vi "Lab Panel V5.0.vi"() -> ()   [LabVIEW 2013] (continued)
                        w1540 = "\\"
                        n878 = local read "SET LAB05-1"() -> (w1548:T5)
                        n879 = case shown="\"CYCLE TEST\"" w1553 {
                          tunnel: ["L05-1-CHART TEST-" "L05-1-CYCLE TEST-" "L05-1-T-RISE TEST-"] -> w1549
                          frame "CHART TEST", Default {
                          }
                          frame "CYCLE TEST" {
                          }
                          frame "T-RISE TEST" {
                          }
                        }
                        n880 = Unbundle(w1548) -> ("DESCRIPTION"=w1547:string)  [unwired: 4 out]
                        n881 = Concatenate Strings(w1543, "\\", w1541, w1540, w1539, w1540) -> (w1550:string)
                        n882 = String To Path(string=w1550) -> (path=w1552:path)
                        n883 = Concatenate Strings(w1550, w1549, w1547, "-", w1546, ".tdms") -> (w1538:string)
                        n884 = Create Folder(path (use dialog)=w1552) -> (error out=w1551:errorcluster)  [unwired: 2 in, 2 out]
                        n885 = global write "Global 1.vi" "LAB05-1 FILE"(w1538) -> ()
                        n886 = call <vilib>:"Clear Errors.vi"("error in (no error)"=w1551) -> ()  [unwired: 6 in, 1 out]
                      }
                      frame #1 {
                        (unwired) FALSE
                        n887 = String To Path(string=w1562) -> (path=w1558:path)
                        n888 = TDMS Open(6:FALSE, 10:T18."create or replace" ("operation (0:open)"), 11:w1558) -> (0:w1557:errorcluster, 3:→"TDMS LAB05-1":refnum<k34>)  [unwired: 4 in]
                      }
                      frame #2 {
                        n889 = local read "SET LAB05-1"() -> (w1568:T5)
                        n890 = local read "TDMS LAB05-1"() -> (w1579:refnum<k34>)
                        n891 = Build Array("Testers Name", "Description", "Set Test Cycles", "T-Rise minutes", "T-Rise Deg C") -> (w1569:string[])
                        n892 = Unbundle(w1568) -> ("NAME"=w1567:string, "DESCRIPTION"=w1566:string, "CYCLES"=w1565:dbl, "T-RISE mins"=w1564:dbl, "T-RISE deg C"=w1563:dbl)
                        n893 = Number To Decimal String(number=w1565) -> (decimal integer string=w1578:string)  [unwired: 1 in]
                        n894 = Number To Decimal String(number=w1564) -> (decimal integer string=w1577:string)  [unwired: 1 in]
                        n895 = Number To Decimal String(number=w1563) -> (decimal integer string=w1576:string)  [unwired: 1 in]
                        n896 = Build Array(w1567, w1566, w1578, w1577, w1576) -> (w1575:string[])
                        n897 = TDMS Set Properties(5:w1575, 7:w1569, 11:w1579) -> ()  [unwired: 3 in, 4 out]
                      }
                      frame #3 {
                        n898 = local read "DISP LAB05-1"() -> (w1584:T4)
                        n899 = Concatenate Strings("LAB05-1  ", w1582) -> (w1585:string)
                        n900 = Two Button Dialog(message=w1585, 1:w1580, 2:w1581) -> (T button?=w1587:bool)
                        n901 = case shown="True" w1587 {
                          tunnel: w1584 -> [w1594 w1595]
                          tunnel: [w1594 w1595] -> w1591
                          tunnel: [w1593 w1596] -> w1590
                          tunnel: [w1592 w1596] -> w1589
                          frame False {
                            n902 = Unbundle(w1594) -> ("CYCLE"=w1593:dbl, "MINS"=w1592:dbl)  [unwired: 1 out]
                          }
                          frame True {
                            w1596 = 0.0
                          }
                        }
                        n903 = Bundle(cluster=w1591, "CYCLE"=w1590, "MINS"=w1589, "STATUS"="RUN") -> (w1583:T4)
                        n904 = local write "DISP LAB05-1"(w1583) -> ()
                      }
                      frame #4 {
                        n905 = local read "SIG LAB05-1"() -> (w1599:T2)
                        n906 = local read "TEMP START LAB05-1"() -> (w1601:cluster{"TL":dbl, "TN":dbl})
                        n907 = Unbundle(w1599) -> ("Tmp Live"=w1598:dbl, "Tmp Neut"=w1597:dbl)  [unwired: 3 out]
                        n908 = Bundle(cluster=w1601, "TL"=w1598, "TN"=w1597) -> (w1600:cluster{"TL":dbl, "TN":dbl})
                        n909 = local write "TEMP START LAB05-1"(w1600) -> ()
                      }
                    }
                  }
                }
              }
              event "RUN LAB05-2": Value Change {
                n910 = event-data() -> ("NewVal"=w1605:bool)  [unwired: 1 in, 5 out]
                n911 = local write "run lab05-2"(w1605) -> ()
                n912 = case shown="True" w1605 {
                  tunnel: w1611 -> [_ w1647]
                  tunnel: w1610 -> [_ w1646]
                  tunnel: w1608 -> [w1613 w1645]
                  tunnel: w1609 -> [_ w1644]
                  tunnel: w1607 -> [_ w1643]
                  tunnel: [w1612 w1642] -> w1606
                  tunnel: w1604 -> [_ w1641]
                  tunnel: w1603 -> [_ w1640]
                  tunnel: w1602 -> [_ w1639]
                  frame False {
                    # "stop test"
                    n913 = stacked-sequence {
                      tunnel: w1613 -> [w1622 _]
                      tunnel: [w1614 _] -> w1612
                      frame #0 {
                        n914 = local read "DISP LAB05-2"() -> (w1621:T4)
                        n915 = Unbundle(w1621) -> ("CYCLE"=w1619:dbl, "MINS"=w1620:dbl)  [unwired: 1 out]
                        n916 = case shown="\"CYCLE TEST\"" w1622 {
                          tunnel: w1620 -> [_ _ w1629]
                          tunnel: w1619 -> [w1627 w1628 _]
                          tunnel: [w1627 w1628 w1629] -> w1618
                          frame "CHART TEST", Default {
                          }
                          frame "CYCLE TEST" {
                          }
                          frame "T-RISE TEST" {
                          }
                        }
                        n917 = local read "TDMS LAB05-2"() -> (w1626:refnum<k34>)
                        n918 = Build Array("STOPPED") -> (w1623:string[])
                        n919 = Build Array(w1618) -> (w1617:dbl[])
                        n920 = TDMS Write(0:w1626, 5:"TEST RESULT", 7:w1623, 9:w1617) -> (4:w1615:refnum<k34>, 15:w1616:errorcluster)  [unwired: 2 in, 2 out]
                        n921 = TDMS Close(8:w1616, 11:w1615) -> (0:w1614:errorcluster)  [unwired: 1 out]
                      }
                      frame #1 {
                        n922 = local read "DISP LAB05-2"() -> (w1633:T4)
                        n923 = stacked-sequence {
                          tunnel: "LAB05-2" -> [w1635 w1637]
                          frame #0 {
                            n924 = call "sub vi - defrag tdms v1.vi"("panel id"=w1635) -> ("error out"=w1634:errorcluster)  [unwired: 10 in]
                            n925 = local write "data file error"(w1634) -> ()
                          }
                          frame #1 {
                            n926 = local write "RESULT LAB05-2"(FALSE) -> ()
                            n927 = call "Save data file to network drive v2.vi"("panel id"=w1637) -> ("network file save error"=w1636:errorcluster)  [unwired: 9 in, 1 out]
                            n928 = local write "data file error"(w1636) -> ()
                          }
                        }
                        n929 = Bundle(cluster=w1633, "STATUS"="STOP") -> (w1631:T4)  [unwired: 2 in]
                        n930 = local write "DISP LAB05-2"(w1631) -> ()
                      }
                    }
                  }
                  frame True {
                    # "start new test and create test file"
                    n931 = stacked-sequence {
                      seq-local: [w1648 _ _ _ _] -> [_ w1672 _ _ _]
                      tunnel: w1647 -> [w1653 _ _ _ _]
                      tunnel: w1646 -> [w1649 _ _ _ _]
                      tunnel: w1645 -> [w1663 _ _ _ _]
                      tunnel: w1644 -> [w1656 _ _ _ _]
                      tunnel: w1643 -> [w1651 _ _ _ _]
                      tunnel: [_ w1667 _ _ _] -> w1642
                      tunnel: w1641 -> [_ _ _ w1692 _]
                      tunnel: w1640 -> [_ _ _ w1691 _]
                      tunnel: w1639 -> [_ _ _ w1690 _]
                      frame #0 {
                        w1650 = "\\"
                        n932 = local read "SET LAB05-2"() -> (w1658:T5)
                        n933 = case shown="\"CYCLE TEST\"" w1663 {
                          tunnel: ["L05-2-CHART TEST-" "L05-2-CYCLE TEST-" "L05-2-T-RISE TEST-"] -> w1659
                          frame "CHART TEST", Default {
                          }
                          frame "CYCLE TEST" {
                          }
                          frame "T-RISE TEST" {
                          }
                        }
                        n934 = Unbundle(w1658) -> ("DESCRIPTION"=w1657:string)  [unwired: 4 out]
                        n935 = Concatenate Strings(w1653, "\\", w1651, w1650, w1649, w1650) -> (w1660:string)
                        n936 = String To Path(string=w1660) -> (path=w1662:path)
                        n937 = Concatenate Strings(w1660, w1659, w1657, "-", w1656, ".tdms") -> (w1648:string)
                        n938 = Create Folder(path (use dialog)=w1662) -> (error out=w1661:errorcluster)  [unwired: 2 in, 2 out]
                        n939 = global write "Global 1.vi" "LAB05-2 FILE"(w1648) -> ()
                        n940 = call <vilib>:"Clear Errors.vi"("error in (no error)"=w1661) -> ()  [unwired: 6 in, 1 out]
                      }
                      frame #1 {
                        (unwired) FALSE
                        n941 = String To Path(string=w1672) -> (path=w1668:path)
                        n942 = TDMS Open(6:FALSE, 10:T18."create or replace" ("operation (0:open)"), 11:w1668) -> (0:w1667:errorcluster, 3:→"TDMS LAB05-2":refnum<k34>)  [unwired: 4 in]
                      }
                      frame #2 {
                        n943 = local read "SET LAB05-2"() -> (w1678:T5)
                        n944 = local read "TDMS LAB05-2"() -> (w1689:refnum<k34>)
                        n945 = Build Array("Testers Name", "Description", "Set Test Cycles", "T-Rise minutes", "T-Rise Deg C") -> (w1679:string[])
                        n946 = Unbundle(w1678) -> ("NAME"=w1677:string, "DESCRIPTION"=w1676:string, "CYCLES"=w1675:dbl, "T-RISE mins"=w1674:dbl, "T-RISE deg C"=w1673:dbl)
                        n947 = Number To Decimal String(number=w1675) -> (decimal integer string=w1688:string)  [unwired: 1 in]
                        n948 = Number To Decimal String(number=w1674) -> (decimal integer string=w1687:string)  [unwired: 1 in]
                        n949 = Number To Decimal String(number=w1673) -> (decimal integer string=w1686:string)  [unwired: 1 in]
                        n950 = Build Array(w1677, w1676, w1688, w1687, w1686) -> (w1685:string[])
                        n951 = TDMS Set Properties(5:w1685, 7:w1679, 11:w1689) -> ()  [unwired: 3 in, 4 out]
                      }
                      frame #3 {
                        n952 = local read "DISP LAB05-2"() -> (w1694:T4)
                        n953 = Concatenate Strings("LAB05-2  ", w1692) -> (w1695:string)
                        n954 = Two Button Dialog(message=w1695, 1:w1690, 2:w1691) -> (T button?=w1697:bool)
                        n955 = case shown="True" w1697 {
                          tunnel: w1694 -> [w1704 w1705]
                          tunnel: [w1704 w1705] -> w1701
                          tunnel: [w1703 w1706] -> w1700
                          tunnel: [w1702 w1706] -> w1699
                          frame False {
                            n956 = Unbundle(w1704) -> ("CYCLE"=w1703:dbl, "MINS"=w1702:dbl)  [unwired: 1 out]
                          }
                          frame True {
                            w1706 = 0.0
                          }
                        }
                        n957 = Bundle(cluster=w1701, "CYCLE"=w1700, "MINS"=w1699, "STATUS"="RUN") -> (w1693:T4)
                        n958 = local write "DISP LAB05-2"(w1693) -> ()
                      }
                      frame #4 {
                        n959 = local read "SIG LAB05-2"() -> (w1709:T2)
                        n960 = local read "TEMP START LAB05-2"() -> (w1711:cluster{"TL":dbl, "TN":dbl})
                        n961 = Unbundle(w1709) -> ("Tmp Live"=w1708:dbl, "Tmp Neut"=w1707:dbl)  [unwired: 3 out]
                        n962 = Bundle(cluster=w1711, "TL"=w1708, "TN"=w1707) -> (w1710:cluster{"TL":dbl, "TN":dbl})
                        n963 = local write "TEMP START LAB05-2"(w1710) -> ()
                      }
                    }
                  }
                }
              }
            }
            n964 = local write "data file error"(w583) -> ()
          }
          frame #4 {
            # "check if test cycles reached for cycle tests, if so then test pass"
            n965 = stacked-sequence {
              tunnel: w1731 -> [_ _ _ _ _ _ _ _ _ _]
              tunnel: w1730 -> [_ _ _ _ _ _ _ _ _ _]
              tunnel: w1729 -> [_ _ _ _ _ _ _ _ _ _]
              tunnel: w1728 -> [_ _ _ _ _ _ _ _ _ _]
              tunnel: w1727 -> [_ _ _ _ _ _ _ _ _ _]
              tunnel: w1726 -> [_ _ _ _ _ _ _ _ _ _]
              tunnel: w1725 -> [_ _ _ _ _ _ _ _ _ _]
              tunnel: w1724 -> [_ _ _ _ _ _ _ _ _ _]
              tunnel: w1723 -> [_ _ _ _ _ _ _ _ _ _]
              tunnel: w1722 -> [_ _ _ _ _ _ _ _ _ _]
              tunnel: w1721 -> [w1737 _ _ _ _ _ _ _ _ _]
              tunnel: w1720 -> [_ w1772 _ _ _ _ _ _ _ _]
              tunnel: w1719 -> [_ _ w1812 _ _ _ _ _ _ _]
              tunnel: w1718 -> [_ _ _ w1852 _ _ _ _ _ _]
              tunnel: w1717 -> [_ _ _ _ w1892 _ _ _ _ _]
              tunnel: w1716 -> [_ _ _ _ _ w1932 _ _ _ _]
              tunnel: w1715 -> [_ _ _ _ _ _ w1972 _ _ _]
              tunnel: w1714 -> [_ _ _ _ _ _ _ w2012 _ _]
              tunnel: w1713 -> [_ _ _ _ _ _ _ _ w2052 _]
              tunnel: w1712 -> [_ _ _ _ _ _ _ _ _ w2092]
              frame #0 {
                # "LAB01-1"
                n966 = Less?(x=w1737, y=2) -> (x < y?=w1735:bool)
                n967 = local read "DISP LAB01-1"() -> (w1738:T4)
                n968 = Unbundle(w1738) -> ("STATUS"=w1732:string)  [unwired: 2 out]
                n969 = Equal?(x=w1732, y="RUN") -> (x = y?=w1734:bool)
                n970 = And(x=w1734, y=w1735) -> (x .and. y?=w1733:bool)
                n971 = case shown="True" w1733 {
                  tunnel: w1738 -> [_ w1743]
                  tunnel: w1737 -> [_ w1747]
                  frame False {
                  }
                  frame True {
                    n972 = local read "SET LAB01-1"() -> (w1749:T5)
                    n973 = local read "TDMS LAB01-1"() -> (w1742:refnum<k34>)
                    n974 = Unbundle(w1749) -> ("CYCLES"=w1740:dbl, "T-RISE mins"=w1746:dbl)  [unwired: 3 out]
                    n975 = case shown="\"CYCLE TEST\"" w1747 {
                      tunnel: w1746 -> [_ _ w1756]
                      tunnel: [w1751 w1753 w1756] -> w1745
                      tunnel: w1740 -> [w1751 w1753 _]
                      tunnel: ["CHART PASS" "CYCLE PASS" "T-RISE PASS"] -> w1744
                      frame "CHART TEST", Default {
                      }
                      frame "CYCLE TEST" {
                      }
                      frame "T-RISE TEST" {
                      }
                    }
                    n976 = Unbundle(w1743) -> ("CYCLE"=w1748:dbl)  [unwired: 2 out]
                    n977 = Increment(x=w1740) -> (x+1=w1741:dbl)
                    n978 = Greater Or Equal?(x=w1748, y=w1741) -> (x >= y?=w1750:bool)
                    n979 = case shown="True" w1750 {
                      tunnel: w1745 -> [w1760 _]
                      tunnel: w1744 -> [w1759 _]
                      tunnel: w1743 -> [w1758 _]
                      tunnel: w1742 -> [w1757 _]
                      frame True {
                        n980 = stacked-sequence {
                          tunnel: w1760 -> [w1764 _]
                          tunnel: w1759 -> [w1762 w1768]
                          tunnel: w1758 -> [_ w1771]
                          tunnel: w1757 -> [w1761 _]
                          frame #0 {
                            n981 = Build Array(w1762) -> (w1765:string[])
                            n982 = Build Array(w1764) -> (w1763:dbl[])
                            n983 = TDMS Write(0:w1761, 5:"TEST PASS", 7:w1765, 9:w1763) -> (15:w1767:errorcluster)  [unwired: 2 in, 3 out]
                            n984 = local write "data file error"(w1767) -> ()
                          }
                          frame #1 {
                            n985 = Bundle(cluster=w1771, "STATUS"=w1768) -> (w1769:T4)  [unwired: 2 in]
                            n986 = local write "RESULT LAB01-1"(TRUE) -> ()
                            n987 = local write "DISP LAB01-1"(w1769) -> ()
                          }
                        }
                      }
                      frame False {
                      }
                    }
                  }
                }
              }
              frame #1 {
                # "LAB01-2"
                n988 = Less?(x=w1772, y=2) -> (x < y?=w1775:bool)
                n989 = local read "DISP LAB01-2"() -> (w1777:T4)
                n990 = Unbundle(w1777) -> ("STATUS"=w1778:string)  [unwired: 2 out]
                n991 = Equal?(x=w1778, y="RUN") -> (x = y?=w1774:bool)
                n992 = And(x=w1774, y=w1775) -> (x .and. y?=w1773:bool)
                n993 = case shown="True" w1773 {
                  tunnel: w1777 -> [_ w1783]
                  tunnel: w1772 -> [_ w1787]
                  frame False {
                  }
                  frame True {
                    n994 = local read "SET LAB01-2"() -> (w1789:T5)
                    n995 = local read "TDMS LAB01-2"() -> (w1782:refnum<k34>)
                    n996 = Unbundle(w1789) -> ("CYCLES"=w1780:dbl, "T-RISE mins"=w1786:dbl)  [unwired: 3 out]
                    n997 = case shown="\"T-RISE TEST\"" w1787 {
                      tunnel: w1786 -> [_ _ w1796]
                      tunnel: [w1791 w1793 w1796] -> w1785
                      tunnel: w1780 -> [w1791 w1793 _]
                      tunnel: ["CHART PASS" "CYCLE PASS" "T-RISE PASS"] -> w1784
                      frame "CHART TEST", Default {
                      }
                      frame "CYCLE TEST" {
                      }
                      frame "T-RISE TEST" {
                      }
                    }
                    n998 = Unbundle(w1783) -> ("CYCLE"=w1788:dbl)  [unwired: 2 out]
                    n999 = Increment(x=w1780) -> (x+1=w1781:dbl)
                    n1000 = Greater Or Equal?(x=w1788, y=w1781) -> (x >= y?=w1790:bool)
                    n1001 = case shown="True" w1790 {
                      tunnel: w1785 -> [w1800 _]
                      tunnel: w1784 -> [w1799 _]
                      tunnel: w1783 -> [w1798 _]
                      tunnel: w1782 -> [w1797 _]
                      frame True {
                        n1002 = stacked-sequence {
                          tunnel: w1800 -> [w1804 _]
                          tunnel: w1799 -> [w1802 w1808]
                          tunnel: w1798 -> [_ w1811]
                          tunnel: w1797 -> [w1801 _]
                          frame #0 {
                            n1003 = Build Array(w1802) -> (w1805:string[])
                            n1004 = Build Array(w1804) -> (w1803:dbl[])
                            n1005 = TDMS Write(0:w1801, 5:"TEST PASS", 7:w1805, 9:w1803) -> (15:w1807:errorcluster)  [unwired: 2 in, 3 out]
                            n1006 = local write "data file error"(w1807) -> ()
                          }
                          frame #1 {
                            n1007 = Bundle(cluster=w1811, "STATUS"=w1808) -> (w1809:T4)  [unwired: 2 in]
                            n1008 = local write "RESULT LAB01-2"(TRUE) -> ()
                            n1009 = local write "DISP LAB01-2"(w1809) -> ()
                          }
                        }
                      }
                      frame False {
                      }
                    }
                  }
                }
              }
              frame #2 {
                # "LAB02-1"
                n1010 = Less?(x=w1812, y=2) -> (x < y?=w1815:bool)
                n1011 = local read "DISP LAB02-1"() -> (w1817:T4)
                n1012 = Unbundle(w1817) -> ("STATUS"=w1818:string)  [unwired: 2 out]
                n1013 = Equal?(x=w1818, y="RUN") -> (x = y?=w1814:bool)
                n1014 = And(x=w1814, y=w1815) -> (x .and. y?=w1813:bool)
                n1015 = case shown="True" w1813 {
                  tunnel: w1817 -> [_ w1823]
                  tunnel: w1812 -> [_ w1827]
                  frame False {
                  }
                  frame True {
                    n1016 = local read "SET LAB02-1"() -> (w1829:T5)
                    n1017 = local read "TDMS LAB02-1"() -> (w1822:refnum<k34>)
                    n1018 = Unbundle(w1823) -> ("CYCLE"=w1828:dbl)  [unwired: 2 out]
                    n1019 = Unbundle(w1829) -> ("CYCLES"=w1820:dbl, "T-RISE mins"=w1826:dbl)  [unwired: 3 out]
                    n1020 = case shown="\"T-RISE TEST\"" w1827 {
                      tunnel: w1826 -> [_ _ w1836]
                      tunnel: [w1831 w1833 w1836] -> w1825
                      tunnel: w1820 -> [w1831 w1833 _]
                      tunnel: ["CHART PASS" "CYCLE PASS" "T-RISE PASS"] -> w1824
                      frame "CHART TEST", Default {
                      }
                      frame "CYCLE TEST" {
                      }
                      frame "T-RISE TEST" {
                      }
                    }
                    n1021 = Increment(x=w1820) -> (x+1=w1821:dbl)
                    n1022 = Greater Or Equal?(x=w1828, y=w1821) -> (x >= y?=w1830:bool)
                    n1023 = case shown="True" w1830 {
                      tunnel: w1825 -> [w1840 _]
                      tunnel: w1824 -> [w1839 _]
                      tunnel: w1823 -> [w1838 _]
                      tunnel: w1822 -> [w1837 _]
                      frame True {
                        n1024 = stacked-sequence {
                          tunnel: w1840 -> [w1844 _]
                          tunnel: w1839 -> [w1842 w1848]
                          tunnel: w1838 -> [_ w1851]
                          tunnel: w1837 -> [w1841 _]
                          frame #0 {
                            n1025 = Build Array(w1842) -> (w1845:string[])
                            n1026 = Build Array(w1844) -> (w1843:dbl[])
                            n1027 = TDMS Write(0:w1841, 5:"TEST PASS", 7:w1845, 9:w1843) -> (15:w1847:errorcluster)  [unwired: 2 in, 3 out]
                            n1028 = local write "data file error"(w1847) -> ()
                          }
                          frame #1 {
                            n1029 = Bundle(cluster=w1851, "STATUS"=w1848) -> (w1849:T4)  [unwired: 2 in]
                            n1030 = local write "RESULT LAB02-1"(TRUE) -> ()
                            n1031 = local write "DISP LAB02-1"(w1849) -> ()
                          }
                        }
                      }
                      frame False {
                      }
                    }
                  }
                }
              }
              frame #3 {
                # "LAB02-2"
                n1032 = Less?(x=w1852, y=2) -> (x < y?=w1855:bool)
                n1033 = local read "DISP LAB02-2"() -> (w1857:T4)
                n1034 = Unbundle(w1857) -> ("STATUS"=w1858:string)  [unwired: 2 out]
                n1035 = Equal?(x=w1858, y="RUN") -> (x = y?=w1854:bool)
                n1036 = And(x=w1854, y=w1855) -> (x .and. y?=w1853:bool)
                n1037 = case shown="True" w1853 {
                  tunnel: w1857 -> [_ w1863]
                  tunnel: w1852 -> [_ w1867]
                  frame False {
                  }
                  frame True {
                    n1038 = local read "SET LAB02-2"() -> (w1869:T5)
                    n1039 = local read "TDMS LAB02-2"() -> (w1862:refnum<k34>)
                    n1040 = Unbundle(w1863) -> ("CYCLE"=w1868:dbl)  [unwired: 2 out]
                    n1041 = Unbundle(w1869) -> ("CYCLES"=w1860:dbl, "T-RISE mins"=w1866:dbl)  [unwired: 3 out]
                    n1042 = case shown="\"T-RISE TEST\"" w1867 {
                      tunnel: w1866 -> [_ _ w1876]
                      tunnel: [w1871 w1873 w1876] -> w1865
                      tunnel: w1860 -> [w1871 w1873 _]
                      tunnel: ["CHART PASS" "CYCLE PASS" "T-RISE PASS"] -> w1864
                      frame "CHART TEST", Default {
                      }
                      frame "CYCLE TEST" {
                      }
                      frame "T-RISE TEST" {
                      }
                    }
                    n1043 = Increment(x=w1860) -> (x+1=w1861:dbl)
                    n1044 = Greater Or Equal?(x=w1868, y=w1861) -> (x >= y?=w1870:bool)
                    n1045 = case shown="True" w1870 {
                      tunnel: w1865 -> [w1880 _]
                      tunnel: w1864 -> [w1879 _]
                      tunnel: w1863 -> [w1878 _]
                      tunnel: w1862 -> [w1877 _]
                      frame True {
                        n1046 = stacked-sequence {
                          tunnel: w1880 -> [w1884 _]
                          tunnel: w1879 -> [w1882 w1888]
                          tunnel: w1878 -> [_ w1891]
                          tunnel: w1877 -> [w1881 _]
                          frame #0 {
                            n1047 = Build Array(w1882) -> (w1885:string[])
                            n1048 = Build Array(w1884) -> (w1883:dbl[])
                            n1049 = TDMS Write(0:w1881, 5:"TEST PASS", 7:w1885, 9:w1883) -> (15:w1887:errorcluster)  [unwired: 2 in, 3 out]
                            n1050 = local write "data file error"(w1887) -> ()
                          }
                          frame #1 {
                            n1051 = Bundle(cluster=w1891, "STATUS"=w1888) -> (w1889:T4)  [unwired: 2 in]
                            n1052 = local write "RESULT LAB02-2"(TRUE) -> ()
                            n1053 = local write "DISP LAB02-2"(w1889) -> ()
                          }
                        }
                      }
                      frame False {
                      }
                    }
                  }
                }
              }
              frame #4 {
                # "LAB03-1"
                n1054 = Less?(x=w1892, y=2) -> (x < y?=w1895:bool)
                n1055 = local read "DISP LAB03-1"() -> (w1897:T4)
                n1056 = Unbundle(w1897) -> ("STATUS"=w1898:string)  [unwired: 2 out]
                n1057 = Equal?(x=w1898, y="RUN") -> (x = y?=w1894:bool)
                n1058 = And(x=w1894, y=w1895) -> (x .and. y?=w1893:bool)
                n1059 = case shown="True" w1893 {
                  tunnel: w1897 -> [_ w1903]
                  tunnel: w1892 -> [_ w1907]
                  frame False {
                  }
                  frame True {
                    n1060 = local read "SET LAB03-1"() -> (w1909:T5)
                    n1061 = local read "TDMS LAB03-1"() -> (w1902:refnum<k34>)
                    n1062 = Unbundle(w1903) -> ("CYCLE"=w1908:dbl)  [unwired: 2 out]
                    n1063 = Unbundle(w1909) -> ("CYCLES"=w1900:dbl, "T-RISE mins"=w1906:dbl)  [unwired: 3 out]
                    n1064 = case shown="\"T-RISE TEST\"" w1907 {
                      tunnel: w1906 -> [_ _ w1916]
                      tunnel: [w1911 w1913 w1916] -> w1905
                      tunnel: w1900 -> [w1911 w1913 _]
                      tunnel: ["CHART PASS" "CYCLE PASS" "T-RISE PASS"] -> w1904
                      frame "CHART TEST", Default {
                      }
                      frame "CYCLE TEST" {
                      }
                      frame "T-RISE TEST" {
                      }
                    }
                    n1065 = Increment(x=w1900) -> (x+1=w1901:dbl)
                    n1066 = Greater Or Equal?(x=w1908, y=w1901) -> (x >= y?=w1910:bool)
                    n1067 = case shown="True" w1910 {
                      tunnel: w1905 -> [w1920 _]
                      tunnel: w1904 -> [w1919 _]
                      tunnel: w1903 -> [w1918 _]
                      tunnel: w1902 -> [w1917 _]
                      frame True {
                        n1068 = stacked-sequence {
                          tunnel: w1920 -> [w1924 _]
                          tunnel: w1919 -> [w1922 w1928]
                          tunnel: w1918 -> [_ w1931]
                          tunnel: w1917 -> [w1921 _]
                          frame #0 {
                            n1069 = Build Array(w1922) -> (w1925:string[])
                            n1070 = Build Array(w1924) -> (w1923:dbl[])
                            n1071 = TDMS Write(0:w1921, 5:"TEST PASS", 7:w1925, 9:w1923) -> (15:w1927:errorcluster)  [unwired: 2 in, 3 out]
                            n1072 = local write "data file error"(w1927) -> ()
                          }
                          frame #1 {
                            n1073 = Bundle(cluster=w1931, "STATUS"=w1928) -> (w1929:T4)  [unwired: 2 in]
                            n1074 = local write "RESULT LAB03-1"(TRUE) -> ()
                            n1075 = local write "DISP LAB03-1"(w1929) -> ()
                          }
                        }
                      }
                      frame False {
                      }
                    }
                  }
                }
              }
              frame #5 {
                # "LAB03-2"
                n1076 = Less?(x=w1932, y=2) -> (x < y?=w1935:bool)
                n1077 = local read "DISP LAB03-2"() -> (w1937:T4)
                n1078 = Unbundle(w1937) -> ("STATUS"=w1938:string)  [unwired: 2 out]
                n1079 = Equal?(x=w1938, y="RUN") -> (x = y?=w1934:bool)
                n1080 = And(x=w1934, y=w1935) -> (x .and. y?=w1933:bool)
                n1081 = case shown="True" w1933 {
                  tunnel: w1937 -> [_ w1943]
                  tunnel: w1932 -> [_ w1947]
                  frame False {
                  }
                  frame True {
                    n1082 = local read "SET LAB03-2"() -> (w1949:T5)
                    n1083 = local read "TDMS LAB03-2"() -> (w1942:refnum<k34>)
                    n1084 = Unbundle(w1943) -> ("CYCLE"=w1948:dbl)  [unwired: 2 out]
                    n1085 = Unbundle(w1949) -> ("CYCLES"=w1940:dbl, "T-RISE mins"=w1946:dbl)  [unwired: 3 out]
                    n1086 = case shown="\"T-RISE TEST\"" w1947 {
                      tunnel: w1946 -> [_ _ w1956]
                      tunnel: [w1951 w1953 w1956] -> w1945
                      tunnel: w1940 -> [w1951 w1953 _]
                      tunnel: ["CHART PASS" "CYCLE PASS" "T-RISE PASS"] -> w1944
                      frame "CHART TEST", Default {
                      }
                      frame "CYCLE TEST" {
                      }
                      frame "T-RISE TEST" {
                      }
                    }
                    n1087 = Increment(x=w1940) -> (x+1=w1941:dbl)
                    n1088 = Greater Or Equal?(x=w1948, y=w1941) -> (x >= y?=w1950:bool)
                    n1089 = case shown="True" w1950 {
                      tunnel: w1945 -> [w1960 _]
                      tunnel: w1944 -> [w1959 _]
                      tunnel: w1943 -> [w1958 _]
                      tunnel: w1942 -> [w1957 _]
                      frame True {
                        n1090 = stacked-sequence {
                          tunnel: w1960 -> [w1964 _]
                          tunnel: w1959 -> [w1962 w1968]
                          tunnel: w1958 -> [_ w1971]
                          tunnel: w1957 -> [w1961 _]
                          frame #0 {
                            n1091 = Build Array(w1962) -> (w1965:string[])
                            n1092 = Build Array(w1964) -> (w1963:dbl[])
                            n1093 = TDMS Write(0:w1961, 5:"TEST PASS", 7:w1965, 9:w1963) -> (15:w1967:errorcluster)  [unwired: 2 in, 3 out]
                            n1094 = local write "data file error"(w1967) -> ()
                          }
                          frame #1 {
                            n1095 = Bundle(cluster=w1971, "STATUS"=w1968) -> (w1969:T4)  [unwired: 2 in]
                            n1096 = local write "RESULT LAB03-2"(TRUE) -> ()
                            n1097 = local write "DISP LAB03-2"(w1969) -> ()
                          }
                        }
                      }
                      frame False {
                      }
                    }
                  }
                }
              }
              frame #6 {
                # "LAB04-1"
                n1098 = Less?(x=w1972, y=2) -> (x < y?=w1975:bool)
                n1099 = local read "DISP LAB04-1"() -> (w1977:T4)
                n1100 = Unbundle(w1977) -> ("STATUS"=w1978:string)  [unwired: 2 out]
                n1101 = Equal?(x=w1978, y="RUN") -> (x = y?=w1974:bool)
                n1102 = And(x=w1974, y=w1975) -> (x .and. y?=w1973:bool)
                n1103 = case shown="True" w1973 {
                  tunnel: w1977 -> [_ w1983]
                  tunnel: w1972 -> [_ w1987]
                  frame False {
                  }
                  frame True {
                    n1104 = local read "SET LAB04-1"() -> (w1989:T5)
                    n1105 = local read "TDMS LAB04-1"() -> (w1982:refnum<k34>)
                    n1106 = Unbundle(w1983) -> ("CYCLE"=w1988:dbl)  [unwired: 2 out]
                    n1107 = Unbundle(w1989) -> ("CYCLES"=w1980:dbl, "T-RISE mins"=w1986:dbl)  [unwired: 3 out]
                    n1108 = case shown="\"T-RISE TEST\"" w1987 {
                      tunnel: w1986 -> [_ _ w1996]
                      tunnel: [w1991 w1993 w1996] -> w1985
                      tunnel: w1980 -> [w1991 w1993 _]
                      tunnel: ["CHART PASS" "CYCLE PASS" "T-RISE PASS"] -> w1984
                      frame "CHART TEST", Default {
                      }
                      frame "CYCLE TEST" {
                      }
                      frame "T-RISE TEST" {
                      }
                    }
                    n1109 = Increment(x=w1980) -> (x+1=w1981:dbl)
                    n1110 = Greater Or Equal?(x=w1988, y=w1981) -> (x >= y?=w1990:bool)
                    n1111 = case shown="True" w1990 {
                      tunnel: w1985 -> [w2000 _]
                      tunnel: w1984 -> [w1999 _]
                      tunnel: w1983 -> [w1998 _]
                      tunnel: w1982 -> [w1997 _]
                      frame True {
                        n1112 = stacked-sequence {
                          tunnel: w2000 -> [w2004 _]
                          tunnel: w1999 -> [w2002 w2008]
                          tunnel: w1998 -> [_ w2011]
                          tunnel: w1997 -> [w2001 _]
                          frame #0 {
                            n1113 = Build Array(w2002) -> (w2005:string[])
                            n1114 = Build Array(w2004) -> (w2003:dbl[])
                            n1115 = TDMS Write(0:w2001, 5:"TEST PASS", 7:w2005, 9:w2003) -> (15:w2007:errorcluster)  [unwired: 2 in, 3 out]
                            n1116 = local write "data file error"(w2007) -> ()
                          }
                          frame #1 {
                            n1117 = Bundle(cluster=w2011, "STATUS"=w2008) -> (w2009:T4)  [unwired: 2 in]
                            n1118 = local write "RESULT LAB04-1"(TRUE) -> ()
                            n1119 = local write "DISP LAB04-1"(w2009) -> ()
                          }
                        }
                      }
                      frame False {
                      }
                    }
                  }
                }
              }
              frame #7 {
                # "LAB04-2"
                n1120 = Less?(x=w2012, y=2) -> (x < y?=w2015:bool)
                n1121 = local read "DISP LAB04-2"() -> (w2017:T4)
                n1122 = Unbundle(w2017) -> ("STATUS"=w2018:string)  [unwired: 2 out]
                n1123 = Equal?(x=w2018, y="RUN") -> (x = y?=w2014:bool)
                n1124 = And(x=w2014, y=w2015) -> (x .and. y?=w2013:bool)
                n1125 = case shown="True" w2013 {
                  tunnel: w2017 -> [_ w2023]
                  tunnel: w2012 -> [_ w2027]
                  frame False {
                  }
                  frame True {
                    n1126 = local read "SET LAB04-2"() -> (w2029:T5)
                    n1127 = local read "TDMS LAB04-2"() -> (w2022:refnum<k34>)
                    n1128 = Unbundle(w2023) -> ("CYCLE"=w2028:dbl)  [unwired: 2 out]
                    n1129 = Unbundle(w2029) -> ("CYCLES"=w2020:dbl, "T-RISE mins"=w2026:dbl)  [unwired: 3 out]
                    n1130 = case shown="\"T-RISE TEST\"" w2027 {
                      tunnel: w2026 -> [_ _ w2036]
                      tunnel: [w2031 w2033 w2036] -> w2025
                      tunnel: w2020 -> [w2031 w2033 _]
                      tunnel: ["CHART PASS" "CYCLE PASS" "T-RISE PASS"] -> w2024
                      frame "CHART TEST", Default {
                      }
                      frame "CYCLE TEST" {
                      }
                      frame "T-RISE TEST" {
                      }
                    }
                    n1131 = Increment(x=w2020) -> (x+1=w2021:dbl)
                    n1132 = Greater Or Equal?(x=w2028, y=w2021) -> (x >= y?=w2030:bool)
                    n1133 = case shown="True" w2030 {
                      tunnel: w2025 -> [w2040 _]
                      tunnel: w2024 -> [w2039 _]
                      tunnel: w2023 -> [w2038 _]
                      tunnel: w2022 -> [w2037 _]
                      frame True {
                        n1134 = stacked-sequence {
                          tunnel: w2040 -> [w2044 _]
                          tunnel: w2039 -> [w2042 w2048]
                          tunnel: w2038 -> [_ w2051]
                          tunnel: w2037 -> [w2041 _]
                          frame #0 {
                            n1135 = Build Array(w2042) -> (w2045:string[])
                            n1136 = Build Array(w2044) -> (w2043:dbl[])
                            n1137 = TDMS Write(0:w2041, 5:"TEST PASS", 7:w2045, 9:w2043) -> (15:w2047:errorcluster)  [unwired: 2 in, 3 out]
                            n1138 = local write "data file error"(w2047) -> ()
                          }
                          frame #1 {
                            n1139 = Bundle(cluster=w2051, "STATUS"=w2048) -> (w2049:T4)  [unwired: 2 in]
                            n1140 = local write "RESULT LAB04-2"(TRUE) -> ()
                            n1141 = local write "DISP LAB04-2"(w2049) -> ()
                          }
                        }
                      }
                      frame False {
                      }
                    }
                  }
                }
              }
              frame #8 {
                # "LAB05-1"
                n1142 = Less?(x=w2052, y=2) -> (x < y?=w2055:bool)
                n1143 = local read "DISP LAB05-1"() -> (w2057:T4)
                n1144 = Unbundle(w2057) -> ("STATUS"=w2058:string)  [unwired: 2 out]
                n1145 = Equal?(x=w2058, y="RUN") -> (x = y?=w2054:bool)
                n1146 = And(x=w2054, y=w2055) -> (x .and. y?=w2053:bool)
                n1147 = case shown="True" w2053 {
                  tunnel: w2057 -> [_ w2063]
                  tunnel: w2052 -> [_ w2067]
                  frame False {
                  }
                  frame True {
                    n1148 = local read "SET LAB05-1"() -> (w2069:T5)
                    n1149 = local read "TDMS LAB05-1"() -> (w2062:refnum<k34>)
                    n1150 = Unbundle(w2063) -> ("CYCLE"=w2068:dbl)  [unwired: 2 out]
                    n1151 = Unbundle(w2069) -> ("CYCLES"=w2060:dbl, "T-RISE mins"=w2066:dbl)  [unwired: 3 out]
                    n1152 = case shown="\"T-RISE TEST\"" w2067 {
                      tunnel: w2066 -> [_ _ w2076]
                      tunnel: [w2071 w2073 w2076] -> w2065
                      tunnel: w2060 -> [w2071 w2073 _]
                      tunnel: ["CHART PASS" "CYCLE PASS" "T-RISE PASS"] -> w2064
                      frame "CHART TEST", Default {
                      }
                      frame "CYCLE TEST" {
                      }
                      frame "T-RISE TEST" {
                      }
                    }
                    n1153 = Increment(x=w2060) -> (x+1=w2061:dbl)
                    n1154 = Greater Or Equal?(x=w2068, y=w2061) -> (x >= y?=w2070:bool)
                    n1155 = case shown="True" w2070 {
                      tunnel: w2065 -> [w2080 _]
                      tunnel: w2064 -> [w2079 _]
                      tunnel: w2063 -> [w2078 _]
                      tunnel: w2062 -> [w2077 _]
                      frame True {
                        n1156 = stacked-sequence {
                          tunnel: w2080 -> [w2084 _]
                          tunnel: w2079 -> [w2082 w2088]
                          tunnel: w2078 -> [_ w2091]
                          tunnel: w2077 -> [w2081 _]
                          frame #0 {
                            n1157 = Build Array(w2082) -> (w2085:string[])
                            n1158 = Build Array(w2084) -> (w2083:dbl[])
                            n1159 = TDMS Write(0:w2081, 5:"TEST PASS", 7:w2085, 9:w2083) -> (15:w2087:errorcluster)  [unwired: 2 in, 3 out]
                            n1160 = local write "data file error"(w2087) -> ()
                          }
                          frame #1 {
                            n1161 = Bundle(cluster=w2091, "STATUS"=w2088) -> (w2089:T4)  [unwired: 2 in]
                            n1162 = local write "RESULT LAB05-1"(TRUE) -> ()
                            n1163 = local write "DISP LAB05-1"(w2089) -> ()
                          }
                        }
                      }
                      frame False {
                      }
                    }
                  }
                }
              }
              frame #9 {
                # "LAB05-2"
                n1164 = Less?(x=w2092, y=2) -> (x < y?=w2095:bool)
                n1165 = local read "DISP LAB05-2"() -> (w2097:T4)
                n1166 = Unbundle(w2097) -> ("STATUS"=w2098:string)  [unwired: 2 out]
                n1167 = Equal?(x=w2098, y="RUN") -> (x = y?=w2094:bool)
                n1168 = And(x=w2094, y=w2095) -> (x .and. y?=w2093:bool)
                n1169 = case shown="True" w2093 {
                  tunnel: w2097 -> [_ w2103]
                  tunnel: w2092 -> [_ w2107]
                  frame False {
                  }
                  frame True {
                    n1170 = local read "SET LAB05-2"() -> (w2109:T5)
                    n1171 = local read "TDMS LAB05-2"() -> (w2102:refnum<k34>)
                    n1172 = Unbundle(w2103) -> ("CYCLE"=w2108:dbl)  [unwired: 2 out]
                    n1173 = Unbundle(w2109) -> ("CYCLES"=w2100:dbl, "T-RISE mins"=w2106:dbl)  [unwired: 3 out]
                    n1174 = case shown="\"T-RISE TEST\"" w2107 {
                      tunnel: w2106 -> [_ _ w2116]
                      tunnel: [w2111 w2113 w2116] -> w2105
                      tunnel: w2100 -> [w2111 w2113 _]
                      tunnel: ["CHART PASS" "CYCLE PASS" "T-RISE PASS"] -> w2104
                      frame "CHART TEST", Default {
                      }
                      frame "CYCLE TEST" {
                      }
                      frame "T-RISE TEST" {
                      }
                    }
                    n1175 = Increment(x=w2100) -> (x+1=w2101:dbl)
                    n1176 = Greater Or Equal?(x=w2108, y=w2101) -> (x >= y?=w2110:bool)
                    n1177 = case shown="True" w2110 {
                      tunnel: w2105 -> [w2120 _]
                      tunnel: w2104 -> [w2119 _]
                      tunnel: w2103 -> [w2118 _]
                      tunnel: w2102 -> [w2117 _]
                      frame True {
                        n1178 = stacked-sequence {
                          tunnel: w2120 -> [w2124 _]
                          tunnel: w2119 -> [w2122 w2128]
                          tunnel: w2118 -> [_ w2131]
                          tunnel: w2117 -> [w2121 _]
                          frame #0 {
                            n1179 = Build Array(w2122) -> (w2125:string[])
                            n1180 = Build Array(w2124) -> (w2123:dbl[])
                            n1181 = TDMS Write(0:w2121, 5:"TEST PASS", 7:w2125, 9:w2123) -> (15:w2127:errorcluster)  [unwired: 2 in, 3 out]
                            n1182 = local write "data file error"(w2127) -> ()
                          }
                          frame #1 {
                            n1183 = Bundle(cluster=w2131, "STATUS"=w2128) -> (w2129:T4)  [unwired: 2 in]
                            n1184 = local write "RESULT LAB05-2"(TRUE) -> ()
                            n1185 = local write "DISP LAB05-2"(w2129) -> ()
                          }
                        }
                      }
                      frame False {
                      }
                    }
                  }
                }
              }
            }
          }
          frame #5 {
            # "check if test cycles reached for temperature rise test"
            n1186 = stacked-sequence {
              tunnel: w2161 -> [_ _ _ _ _ _ _ _ _ _]
              tunnel: w2160 -> [_ _ _ _ _ _ _ _ _ _]
              tunnel: w2159 -> [_ _ _ _ _ _ _ _ _ _]
              tunnel: w2158 -> [_ _ _ _ _ _ _ _ _ _]
              tunnel: w2157 -> [_ _ _ _ _ _ _ _ _ _]
              tunnel: w2156 -> [_ _ _ _ _ _ _ _ _ _]
              tunnel: w2155 -> [_ _ _ _ _ _ _ _ _ _]
              tunnel: w2154 -> [_ _ _ _ _ _ _ _ _ _]
              tunnel: w2153 -> [_ _ _ _ _ _ _ _ _ _]
              tunnel: w2152 -> [_ _ _ _ _ _ _ _ _ _]
              tunnel: w2151 -> [w2167 _ _ _ _ _ _ _ _ _]
              tunnel: w2141 -> [w2162 _ _ _ _ _ _ _ _ _]
              tunnel: w2150 -> [_ w2193 _ _ _ _ _ _ _ _]
              tunnel: w2149 -> [_ _ w2223 _ _ _ _ _ _ _]
              tunnel: w2148 -> [_ _ _ w2253 _ _ _ _ _ _]
              tunnel: w2147 -> [_ _ _ _ w2283 _ _ _ _ _]
              tunnel: w2146 -> [_ _ _ _ _ w2313 _ _ _ _]
              tunnel: w2145 -> [_ _ _ _ _ _ w2343 _ _ _]
              tunnel: w2144 -> [_ _ _ _ _ _ _ w2373 _ _]
              tunnel: w2143 -> [_ _ _ _ _ _ _ _ w2403 _]
              tunnel: w2142 -> [_ _ _ _ _ _ _ _ _ w2433]
              tunnel: w2140 -> [_ w2192 _ _ _ _ _ _ _ _]
              tunnel: w2139 -> [_ _ w2222 _ _ _ _ _ _ _]
              tunnel: w2138 -> [_ _ _ w2252 _ _ _ _ _ _]
              tunnel: w2137 -> [_ _ _ _ w2282 _ _ _ _ _]
              tunnel: w2136 -> [_ _ _ _ _ w2312 _ _ _ _]
              tunnel: w2135 -> [_ _ _ _ _ _ w2342 _ _ _]
              tunnel: w2134 -> [_ _ _ _ _ _ _ w2372 _ _]
              tunnel: w2133 -> [_ _ _ _ _ _ _ _ w2402 _]
              tunnel: w2132 -> [_ _ _ _ _ _ _ _ _ w2432]
              frame #0 {
                # "LAB01-1"
                n1187 = Equal?(x=w2167, y=2) -> (x = y?=w2165:bool)
                n1188 = local read "DISP LAB01-1"() -> (w2168:T4)
                n1189 = Unbundle(w2168) -> ("STATUS"=w2169:string)  [unwired: 2 out]
                n1190 = Equal?(x=w2169, y="RUN") -> (x = y?=w2164:bool)
                n1191 = And(x=w2164, y=w2165) -> (x .and. y?=w2163:bool)
                n1192 = case shown="True" w2163 {
                  tunnel: w2168 -> [_ w2172]
                  tunnel: w2162 -> [_ w2175]
                  frame False {
                  }
                  frame True {
                    n1193 = local read "SET LAB01-1"() -> (w2174:T5)
                    n1194 = local read "TDMS LAB01-1"() -> (w2171:refnum<k34>)
                    n1195 = Unbundle(w2172) -> ("CYCLE"=w2176:dbl)  [unwired: 2 out]
                    n1196 = Unbundle(w2174) -> ("T-RISE mins"=w2173:dbl)  [unwired: 4 out]
                    n1197 = Greater Or Equal?(x=w2176, y=w2175) -> (x >= y?=w2177:bool)
                    n1198 = case shown="True" w2177 {
